vi "ff_retag_device_readdress_retagblocks.vi"(8 "error in (no error)":errorcluster) -> (0 "error out":errorcluster, 1 "new device tag numbers out":i32[](array[numeric]), 2 "error string out.":string, 3 "error retaggin blocks":bool, 5 "error readdressing \ndevices":bool, 7 "error retagging\ndevices":bool)   [LabVIEW 2016]
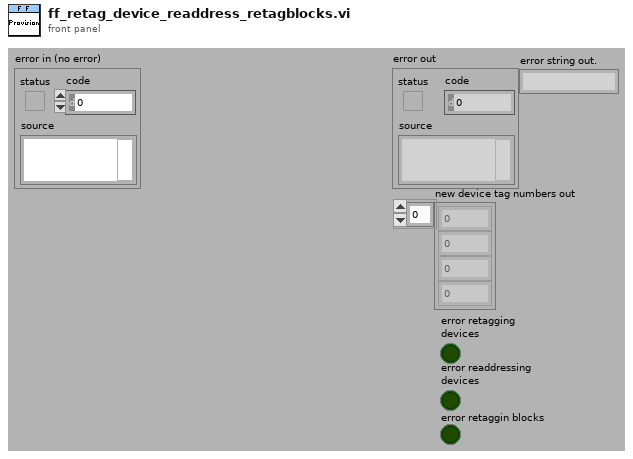
[diagram p1: front panel]
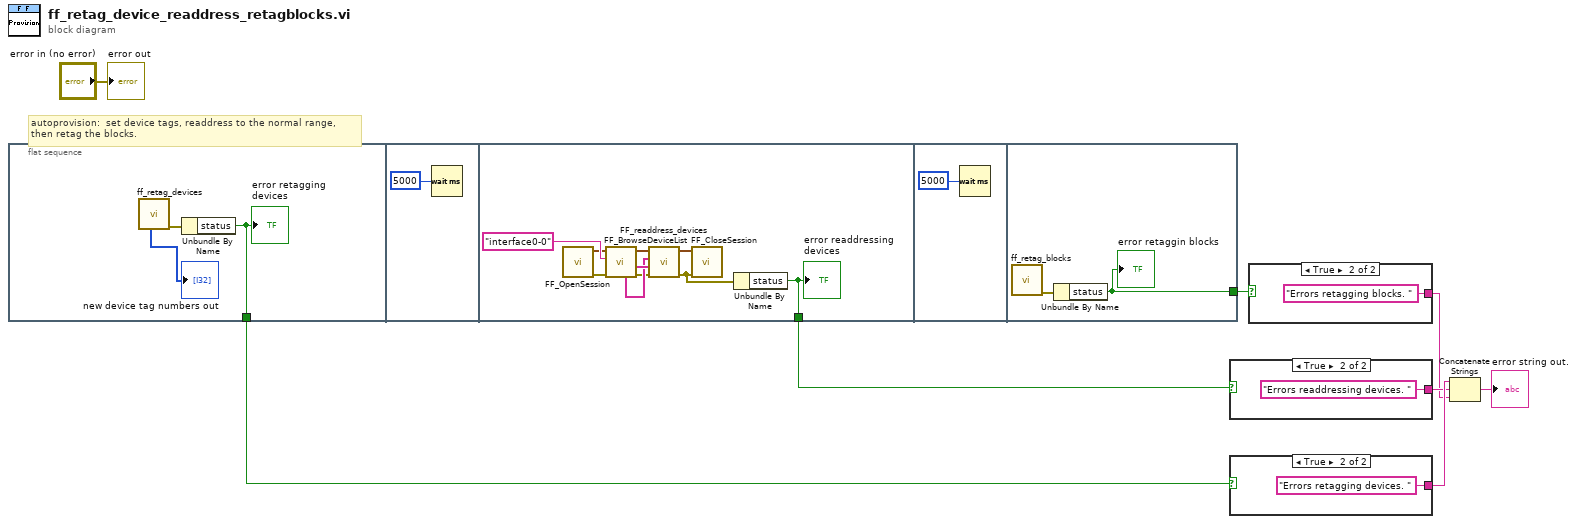
[diagram p0: block diagram]
diagram:
  # "autoprovision:  set device tags, readdress to the normal range, \nthen retag the blocks."
  n1 = flat-sequence {
    tunnel: [w9] -> w7
    tunnel: [w13] -> w6
    tunnel: [w24] -> w1
    frame #0 {
      n2 = call "ff_retag_devices.vi"() -> ("error out"=w10:errorcluster, "new device tag numbers out"=→"new device tag numbers out":i32[])  [unwired: 5 in, 5 out]
      n3 = Unbundle By Name(w10) -> ("status"=w9:bool)
      "error retagging\ndevices" <- w9
    }
    frame #1 {
      n4 = Wait (ms)(milliseconds to wait=u32 5000) -> ()  [unwired: 1 out]
    }
    frame #2 {
      n5 = call "FF_OpenSession.vi"() -> ("error out"=w17:errorcluster, "refnum out"=w16:cluster{"Handle1":u32, "Handle2":u32})  [unwired: 10 in]
      n6 = call "FF_BrowseDeviceList.vi"("error in (no error)"=w17, "link name"="interface0-0", "refnum in"=w16) -> ("error out"=w14:errorcluster, "deviceID list"=w21:string[], "refnum out"=w19:cluster{"Handle1":u32, "Handle2":u32}, "address list"=w20:string[])  [unwired: 4 in, 1 out]
      n7 = call "FF_readdress_devices.vi"("error in (no error)"=w14, "deviceID list"=w21, "address list"=w20, "refnum in"=w19) -> ("Error Out"=w15:errorcluster, "refnum out"=w22:cluster{"Handle1":u32, "Handle2":u32})  [unwired: 4 in, 2 out]
      n8 = call "FF_CloseSession.vi"("error in (no error)"=w15, "refnum in"=w22) -> ()  [unwired: 9 in, 1 out]
      n9 = Unbundle By Name(w15) -> ("status"=w13:bool)
      "error readdressing \ndevices" <- w13
    }
    frame #3 {
      n10 = Wait (ms)(milliseconds to wait=u32 5000) -> ()  [unwired: 1 out]
    }
    frame #4 {
      n11 = call "ff_retag_blocks.vi"() -> ("error out"=w25:errorcluster)  [unwired: 11 in]
      n12 = Unbundle By Name(w25) -> ("status"=w24:bool)
      "error retaggin blocks" <- w24
    }
  }
  n13 = case shown="True" w6 {
    tunnel: [_ "Errors readdressing devices. "] -> w4
    frame False {
    }
    frame True {
    }
  }
  n14 = case shown="True" w7 {
    tunnel: [_ "Errors retagging devices. "] -> w5
    frame False {
    }
    frame True {
    }
  }
  n15 = case shown="True" w1 {
    tunnel: [_ "Errors retagging blocks. "] -> w3
    frame False {
    }
    frame True {
    }
  }
  n16 = Concatenate Strings(w5, w4, w3) -> (→"error string out.":string)
  "error out" <- "error in (no error)"
